vi "ViewFIFOTrace.vi"() -> ()   [LabVIEW 2009]
panel:
  out "size(s)":i32[](array[numeric])
  in  "binning [ms]":dbl
  in  "stop":bool
  out "MCS Trace":cluster{dbl, dbl, "MCS":u32[][]}(graph)
  in  "line":i32=1 min=1
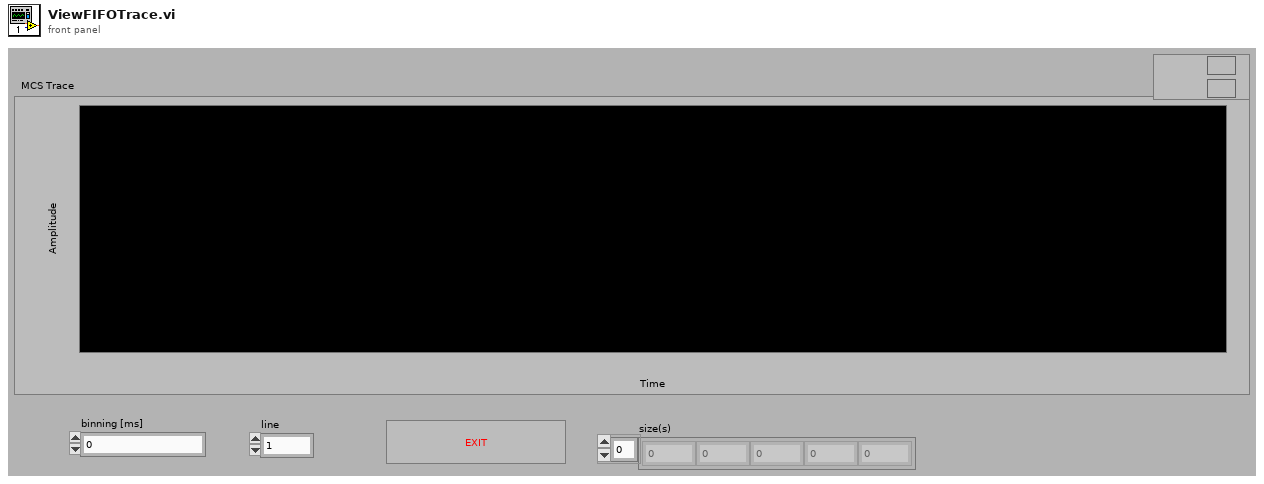
[diagram p1: front panel]
types:
  T1 = cluster{"router":u8[], "macro times":dbl[], "micro times":u16[], "invalid":dbl[], "gap":dbl[]}
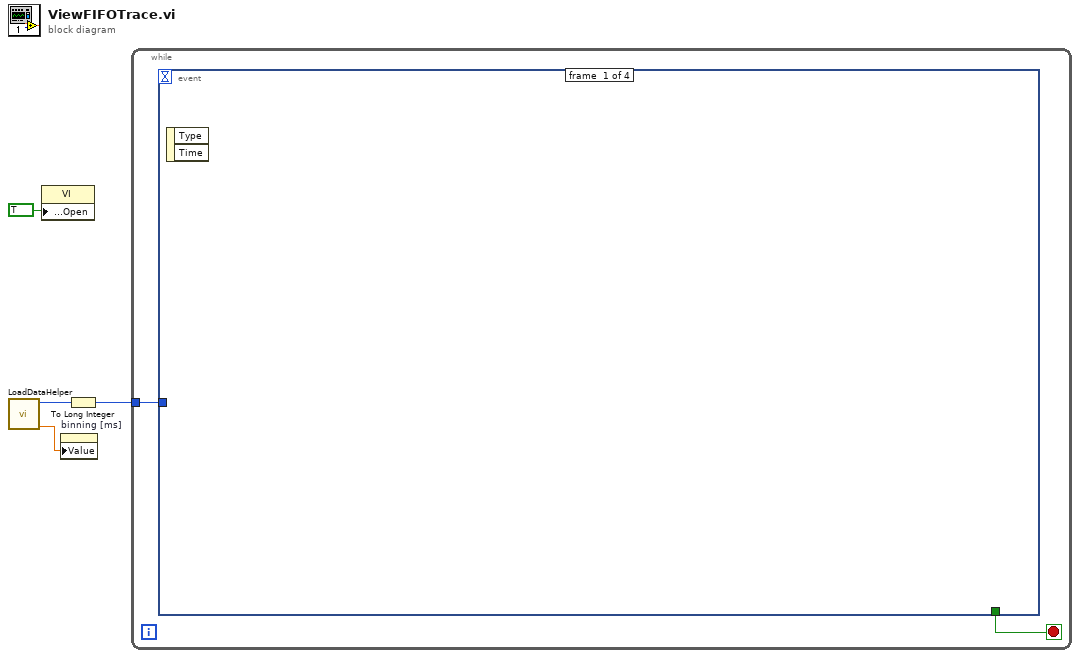
[diagram p0: block diagram]
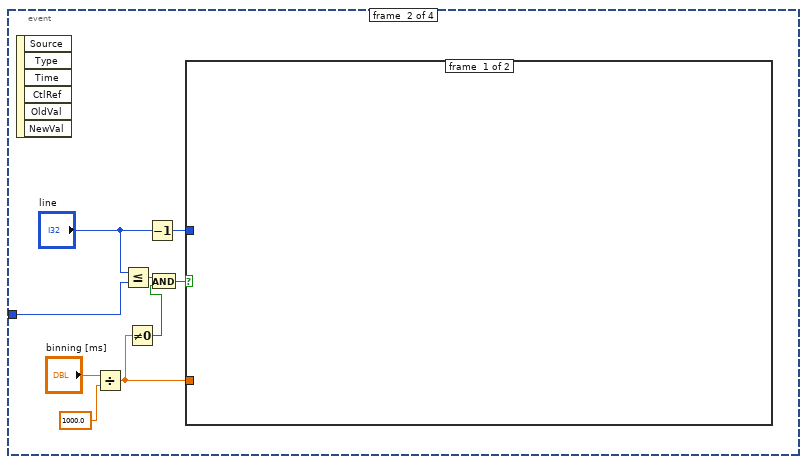
[diagram p2: hidden frame]
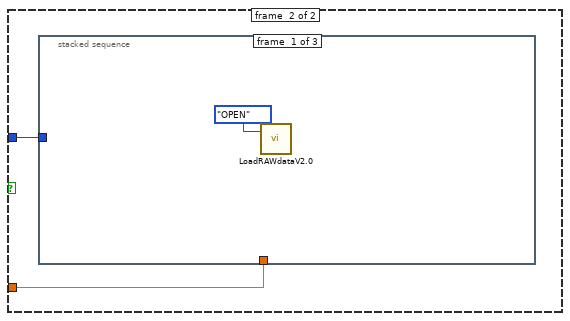
[diagram p3: hidden frame]
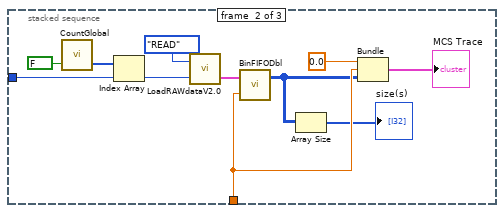
[diagram p4: hidden frame]
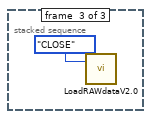
[diagram p5: hidden frame]
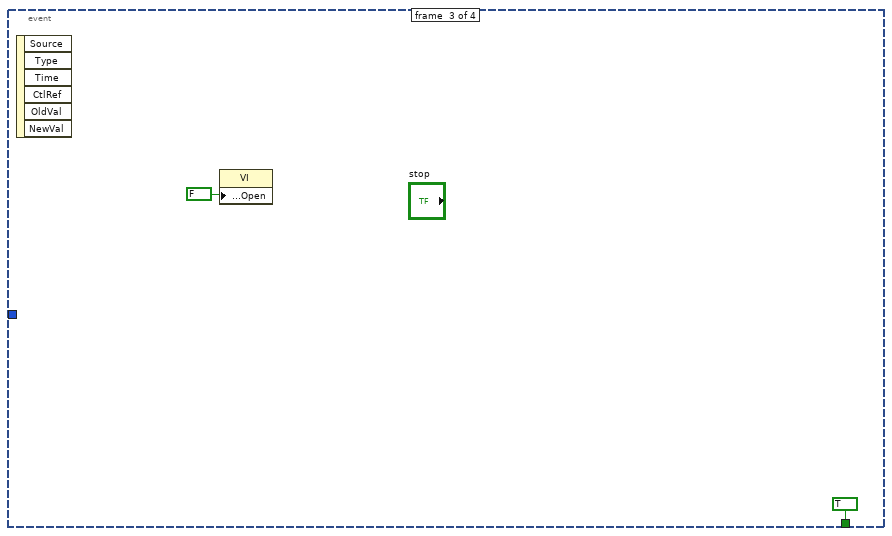
[diagram p6: hidden frame]
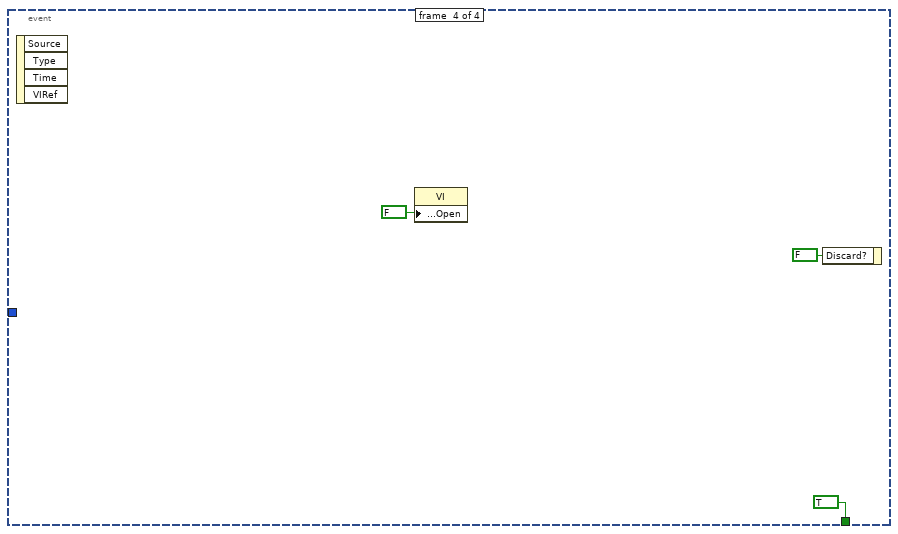
[diagram p7: hidden frame]
diagram:
  n1 = call "LoadDataHelper.vi"() -> ("Time Resolution [ms/pixel]"=w2:dbl, "lines"=w4:u32)  [unwired: 7 in, 3 out]
  n2 = property class="VI"("Front Panel Window:Open"=TRUE) -> ()  [unwired: 2 in, 2 out]
  n3 = property on="binning [ms]" class="DigNum (strict)"("Value"=w2) -> ()  [unwired: 2 in, 2 out]
  n4 = To Long Integer(number=w4) -> (32bit integer=w1:i32)
  n5 = while {
    tunnel: w1 -> [w5]
    stop <- w6 stop-if-true
    n6 = event shown="[1] \"line\", \"binning [ms]\": Value Change" {
      selector: _ -> [_ _ _ _]
      dyn-events: _ -> [_ _ _ _]
      timeout: _ -> [_ _ _ _]
      tunnel: [_ _ TRUE TRUE] -> w6
      tunnel: w5 -> [_ w13 _ _]
      event #0 {
        n7 = event-data() -> ()  [unwired: 1 in, 2 out]
      }
      event #1 {
        n8 = event-data() -> ()  [unwired: 1 in, 6 out]
        n9 = Divide(x="binning [ms]", y=1000.0) -> (x/y=w8:dbl)
        n10 = Less Or Equal?(x="line", y=w13) -> (x <= y?=w10:bool)
        n11 = Not Equal To 0?(x=w8) -> (x != 0?=w7:bool)
        n12 = Decrement(x="line") -> (x-1=w14:i32)
        n13 = And(x=w10, y=w7) -> (x .and. y?=w9:bool)
        n14 = case shown="True" w9 {
          tunnel: w14 -> [_ w17]
          tunnel: w8 -> [_ w16]
          frame #0 {
          }
          frame #1 {
            n15 = stacked-sequence {
              tunnel: w17 -> [_ w29 _]
              tunnel: w16 -> [_ w23 _]
              frame #0 {
                n16 = call "LoadRAWdataV2.0.vi"("action"=enum16{"OPEN", "READ", "CLOSE"}."OPEN" ("Enum")) -> ()  [unwired: 1 in, 2 out]
              }
              frame #1 {
                n17 = call "CountGlobal.vi"("changed?"=FALSE) -> ("count out"=w27:i32[])  [unwired: 2 in]
                n18 = Index Array(array=w27, index=w29) -> (element=w28:i32)
                n19 = call "LoadRAWdataV2.0.vi"("pos offset (0)"=w28, "action"=enum16{"OPEN", "READ", "CLOSE"}."READ" ("Enum")) -> ("RAW data"=w24:T1)  [unwired: 1 out]
                n20 = call "BinFIFODbl.vi"("binning (s)"=w23, "rawdata"=w24) -> ("MCS"=w20:u32[][])  [unwired: 1 out]
                n21 = Array Size(array=w20) -> (size(s)=→"size(s)":i32[])
                n22 = Bundle(0.0, w23, "MCS"=w20) -> (→"MCS Trace":cluster{dbl, dbl, "MCS":u32[][]})  [unwired: 1 in]
              }
              frame #2 {
                n23 = call "LoadRAWdataV2.0.vi"("action"=enum16{"OPEN", "READ", "CLOSE"}."CLOSE" ("Enum")) -> ()  [unwired: 1 in, 2 out]
              }
            }
          }
        }
      }
      event #2 {
        n24 = event-data() -> ()  [unwired: 1 in, 6 out]
        n25 = property class="VI"("Front Panel Window:Open"=FALSE) -> ()  [unwired: 2 in, 2 out]
      }
      event #3 {
        n26 = event-data() -> ()  [unwired: 1 in, 4 out]
        n27 = property class="VI"("Front Panel Window:Open"=FALSE) -> ()  [unwired: 2 in, 2 out]
        n28 = event-data("Discard?"=FALSE) -> ()  [unwired: 1 in, 1 out]
      }
    }
  }
